vi "Sequence_Waveform_Visualizer.vi"() -> ()   [LabVIEW 2010]
panel:
  out "Number of waveforms":i32
  in  "Starting index":i32
  in  "Number to skip":i32=1
  out "Channel 4, \nMarker 1":T1(graph)
  out "Channel 4,\nMarker 2":T1(graph)
  out "Channel 3, \nMarker 1":T1(graph)
  out "Channel 3,\nMarker 2":T1(graph)
  out "Channel 2, \nMarker 1":T1(graph)
  out "Channel 2,\nMarker 2":T1(graph)
  out "Channel 1, \nMarker 1":T1(graph)
  out "Channel 1,\nMarker 2":T1(graph)
  out "Channel 4,\nAnalog":T2(graph)
  out "Channel 3,\nAnalog":T2(graph)
  out "Channel 2,\nAnalog":T2(graph)
  out "Channel 1,\nAnalog":T2(graph)
  in  "stop":bool
  out "Channel Data":sgl[][][](array[numeric])
  out "Marker 1 Data":u8[][][](array[numeric])
  out "Marker 1 Data 2":u8[][][](array[numeric])
  out "error out":errorcluster
  in  "file (use dialog)":path
  in  "error in":errorcluster
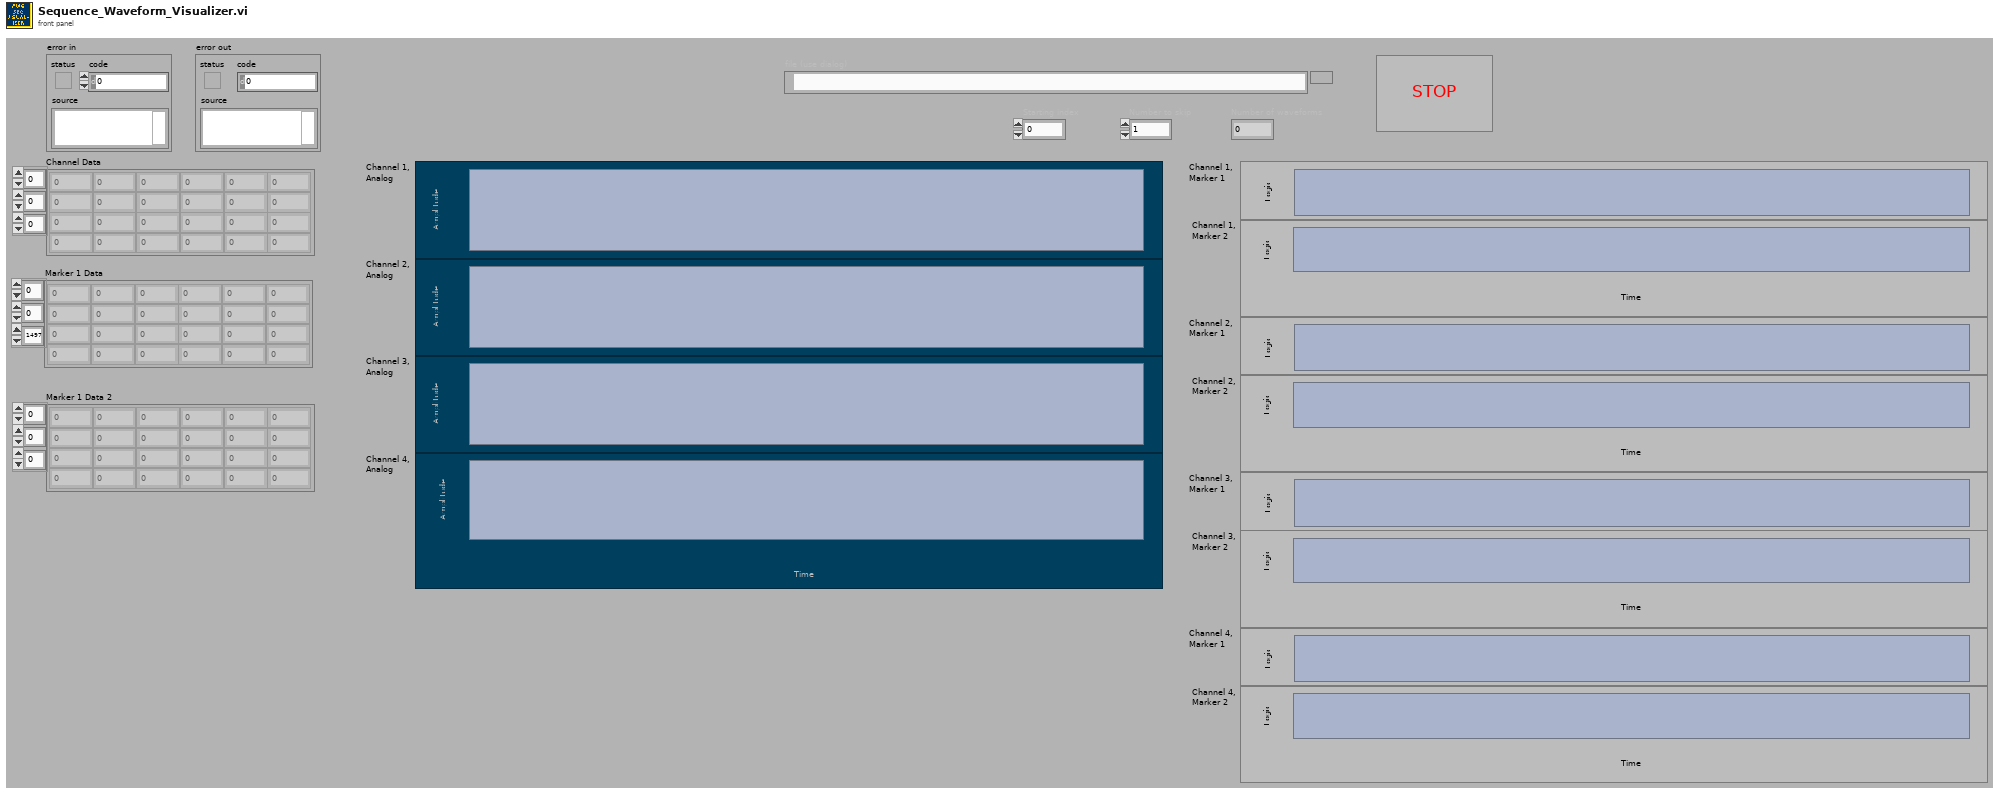
[diagram p1: front panel]
types:
  T1 = cluster{"Sample Period (ns)":dbl, "Sample Period (ns)":dbl, u8[][]}
  T2 = cluster{"Sample Period (ns)":dbl, "Sample Period (ns)":dbl, dbl[][]}
  T3 = cluster{cluster{"Sample Period (ns)":dbl, "Sample Period (ns)":dbl, dbl[][]}, cluster{"Sample Period (ns)":dbl, "Sample Period (ns)":dbl, u8[][]}, cluster{"Sample Period (ns)":dbl, "Sample Period (ns)":dbl, u8[][]}}
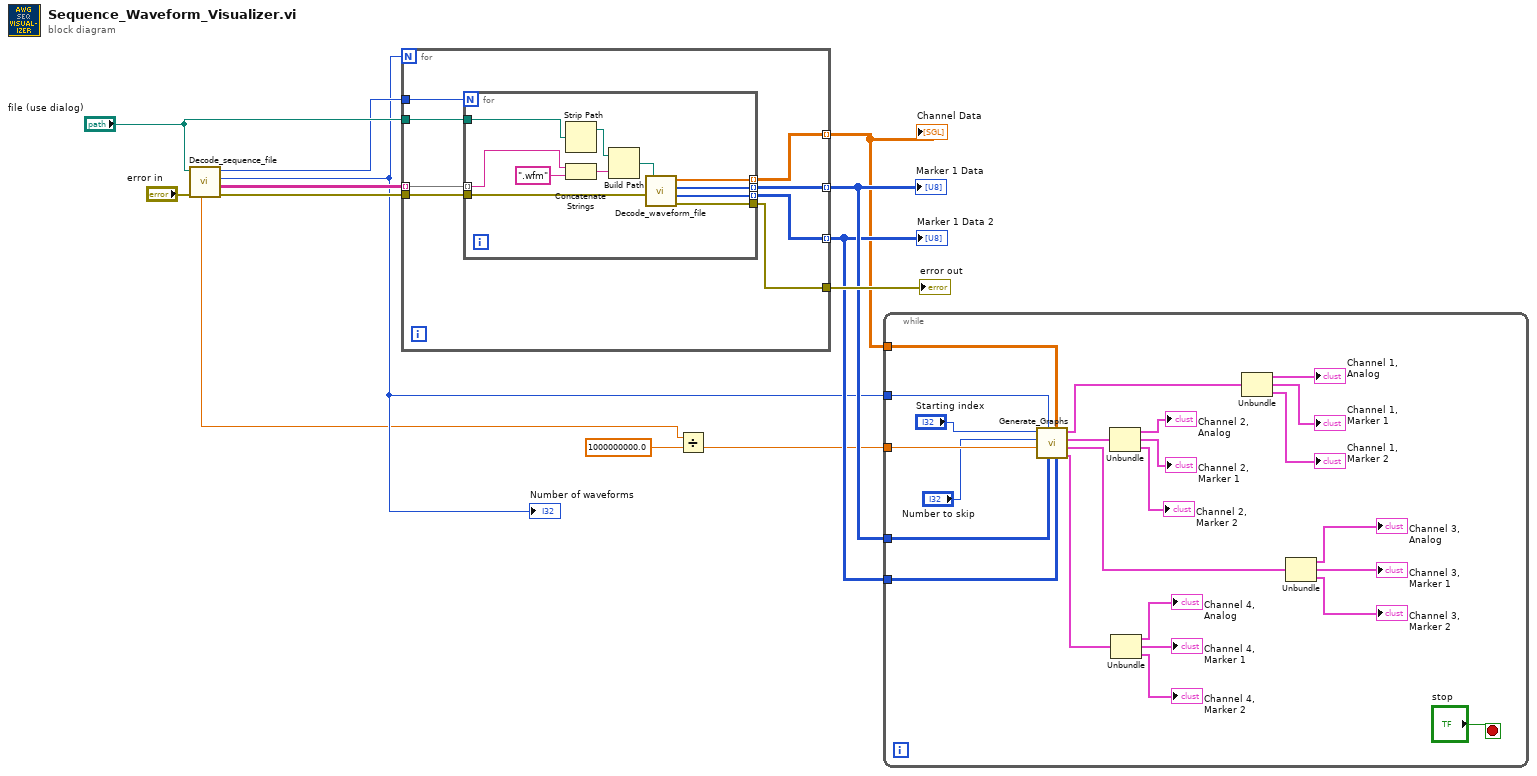
[diagram p0: block diagram]
diagram:
  n1 = call "Decode_sequence_file.vi"("error in"="error in", "file (use dialog)"="file (use dialog)") -> ("error out"=w11:errorcluster, "Waveform Filenames"=w9:string[][], "Number of lines"=w4:i32, "Number of channels"=w10:i32, "Sample Clock"=w2:dbl)  [unwired: 2 in, 1 out]
  "Number of waveforms" <- w4
  n2 = for {
    N: w4 -> [_]
    tunnel: "file (use dialog)" -> [w21]
    tunnel: w11 -> [w20]
    tunnel: w10 -> [w19]
    tunnel: w9 -> [w18] mode=indexing
    tunnel: [w17] -> w5 mode=indexing
    tunnel: [w16] -> w7 mode=indexing
    tunnel: [w15] -> w6 mode=indexing
    tunnel: [w14] -> w8
    n3 = for {
      N: w19 -> [_]
      tunnel: w21 -> [w32]
      tunnel: w20 -> [w27]
      tunnel: w18 -> [w26] mode=indexing
      tunnel: [w25] -> w17 mode=indexing
      tunnel: [w24] -> w16 mode=indexing
      tunnel: [w22] -> w15 mode=indexing
      tunnel: [w23] -> w14
      n4 = Strip Path(path=w32) -> (stripped path=w31:path)  [unwired: 1 out]
      n5 = Concatenate Strings(w26, ".wfm" ("string")) -> (w30:string)
      n6 = Build Path(base path=w31, name or relative path=w30) -> (appended path=w28:path)
      n7 = call "Decode_waveform_file.vi"("error in"=w27, "Waveform file"=w28) -> ("error out"=w23:errorcluster, "Marker 1 Data 2"=w22:u8[], "Marker 1 Data"=w24:u8[], "Channel Data"=w25:sgl[])  [unwired: 2 in]
    }
  }
  "error out" <- w8
  "Marker 1 Data 2" <- w6
  "Marker 1 Data" <- w7
  "Channel Data" <- w5
  n8 = Divide(x=w2, y=1000000000.0) -> (x/y=w3:dbl)
  n9 = while {
    tunnel: w7 -> [w54]
    tunnel: w6 -> [w53]
    tunnel: w5 -> [w55]
    tunnel: w4 -> [w36]
    tunnel: w3 -> [w35]
    stop <- "stop" stop-if-true
    n10 = call "Generate_Graphs.vi"("Marker 1 Data 2"=w53, "Channel Data"=w55, "Marker 1 Data"=w54, "Number of Waveforms"=w36, "Sample Period (ns)"=w35, "Number to skip"="Number to skip", "Starting index"="Starting index") -> ("Chan4"=w37:T3, "Chan3"=w41:T3, "Chan2"=w48:T3, "Chan1"=w52:T3)  [unwired: 1 in]
    n11 = Unbundle(w48) -> (→"Channel 2,\nAnalog":T2, →"Channel 2, \nMarker 1":T1, →"Channel 2,\nMarker 2":T1)
    n12 = Unbundle(w37) -> (→"Channel 4,\nAnalog":T2, →"Channel 4, \nMarker 1":T1, →"Channel 4,\nMarker 2":T1)
    n13 = Unbundle(w52) -> (→"Channel 1,\nAnalog":T2, →"Channel 1, \nMarker 1":T1, →"Channel 1,\nMarker 2":T1)
    n14 = Unbundle(w41) -> (→"Channel 3,\nAnalog":T2, →"Channel 3, \nMarker 1":T1, →"Channel 3,\nMarker 2":T1)
  }
